vi "Test-TestIntake.vi"() -> ()   [LabVIEW 2023]
doc: "This VI implements the framework and scheduler for your robotics program. It should not be necessary to modify the framework. You are expected to add your code to the VIs called from Robot Main - the ones located in the Team Code folder within the project."
uses:
  <vilib>/Rock Robotics/WPI/DriverStation/WPI_DriverStationRobotMode2.ctl
  Intake/IntakeStates.ctl
  Robot Global Data.vi
  Intake/IntakeCancelSendCmd.vi
  Intake/IntakeAlgaeSendCmd.vi
  Intake/IntakeDepositAlgaeSendCmd.vi
  Intake/IntakeCoralSendCmd.vi
  Intake/IntakeDepositCoralSendCmd.vi
  <vilib>/Rock Robotics/WPI/ThirdParty/JAS_Junk/TrajLib/Trajectory_Library.lvlib
panel:
  out "Numeric":i32
  out "CurrentState":T1
  in  "HaveAlgae":bool
  in  "HaveCoral":bool
  out "Waveform Chart":T2(graph)
  out "Right Motor Out":dbl format="%9.1f"
  in  "IntakeCoral":bool
  in  "CmdSpecific":bool
  in  "Specific":dbl
  in  "IntakeAlgae":bool
  out "Left Motor Out":dbl format="%9.1f"
  in  "DepositCoral":bool
  in  "DepositAlgae":bool
  in  "Canel":bool
  out "Robot Mode":T3
  out "Top Motor Out":dbl format="%9.2f"
  in  "error in (no error)":errorcluster
  in  "Finish":bool
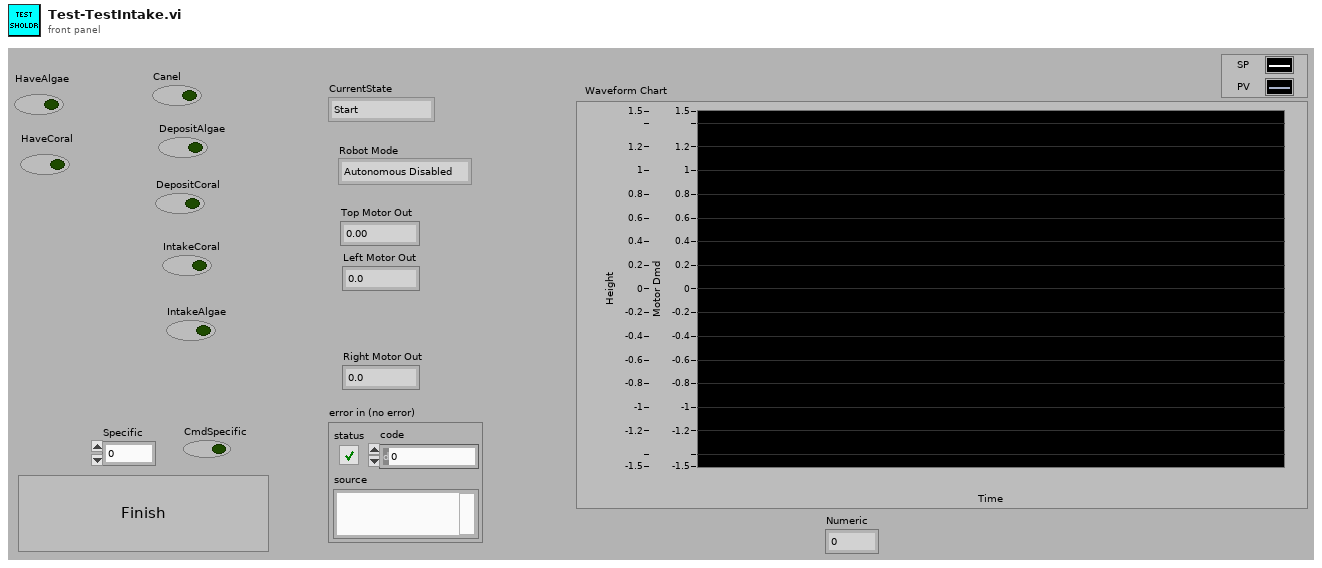
[diagram p1: front panel]
types:
  T1 = typedef "IntakeStates.ctl" = enum16{"Start", "WaitForCommand", "IntakeCoral", "IntakeAlgae", "WaitForCoral", "WaitForAlgae", "DepositCoral", "DepositAlgae", "DepositCoralTimer", "DepositAlgaeTimer"}
  T2 = cluster{"ElevatorPosDemandHeight":dbl, "ElevHeightInch":dbl, "MotorDemand":dbl}
  T3 = typedef "WPI_DriverStationRobotMode2.ctl" = enum16{"Autonomous Disabled", "Autonomous Enabled", "Teleop Disabled", "Teleop Enabled", "Disconnected", "Finish", "Test Disabled", "Test Enabled", "Emergency Stopped"}
  T4 = cluster{"MotorDemandTop":dbl, "MotorDemandLeft":dbl, "MotorDemandRight":dbl}
  T5 = typedef "WPI_DriverStationMatch Info.ctl" = cluster{"Autonomous Elapsed Seconds":dbl, "TeleOp Elapsed Seconds":dbl, "Disabled Elapsed Seconds":dbl, "Visited Autonomous":bool, "Visited TeleOp":bool, "Visited Disabled":bool, "Autonomous Settings":cluster{"Autonomous Style":enum16{"Iterative", "Independent"}, "VI Refnum":refnum<vi>}}
  T6 = typedef "WPI_DriverStationDerivedRobotMode.ctl" = enum16{"Init", "Execute", "Stop"}
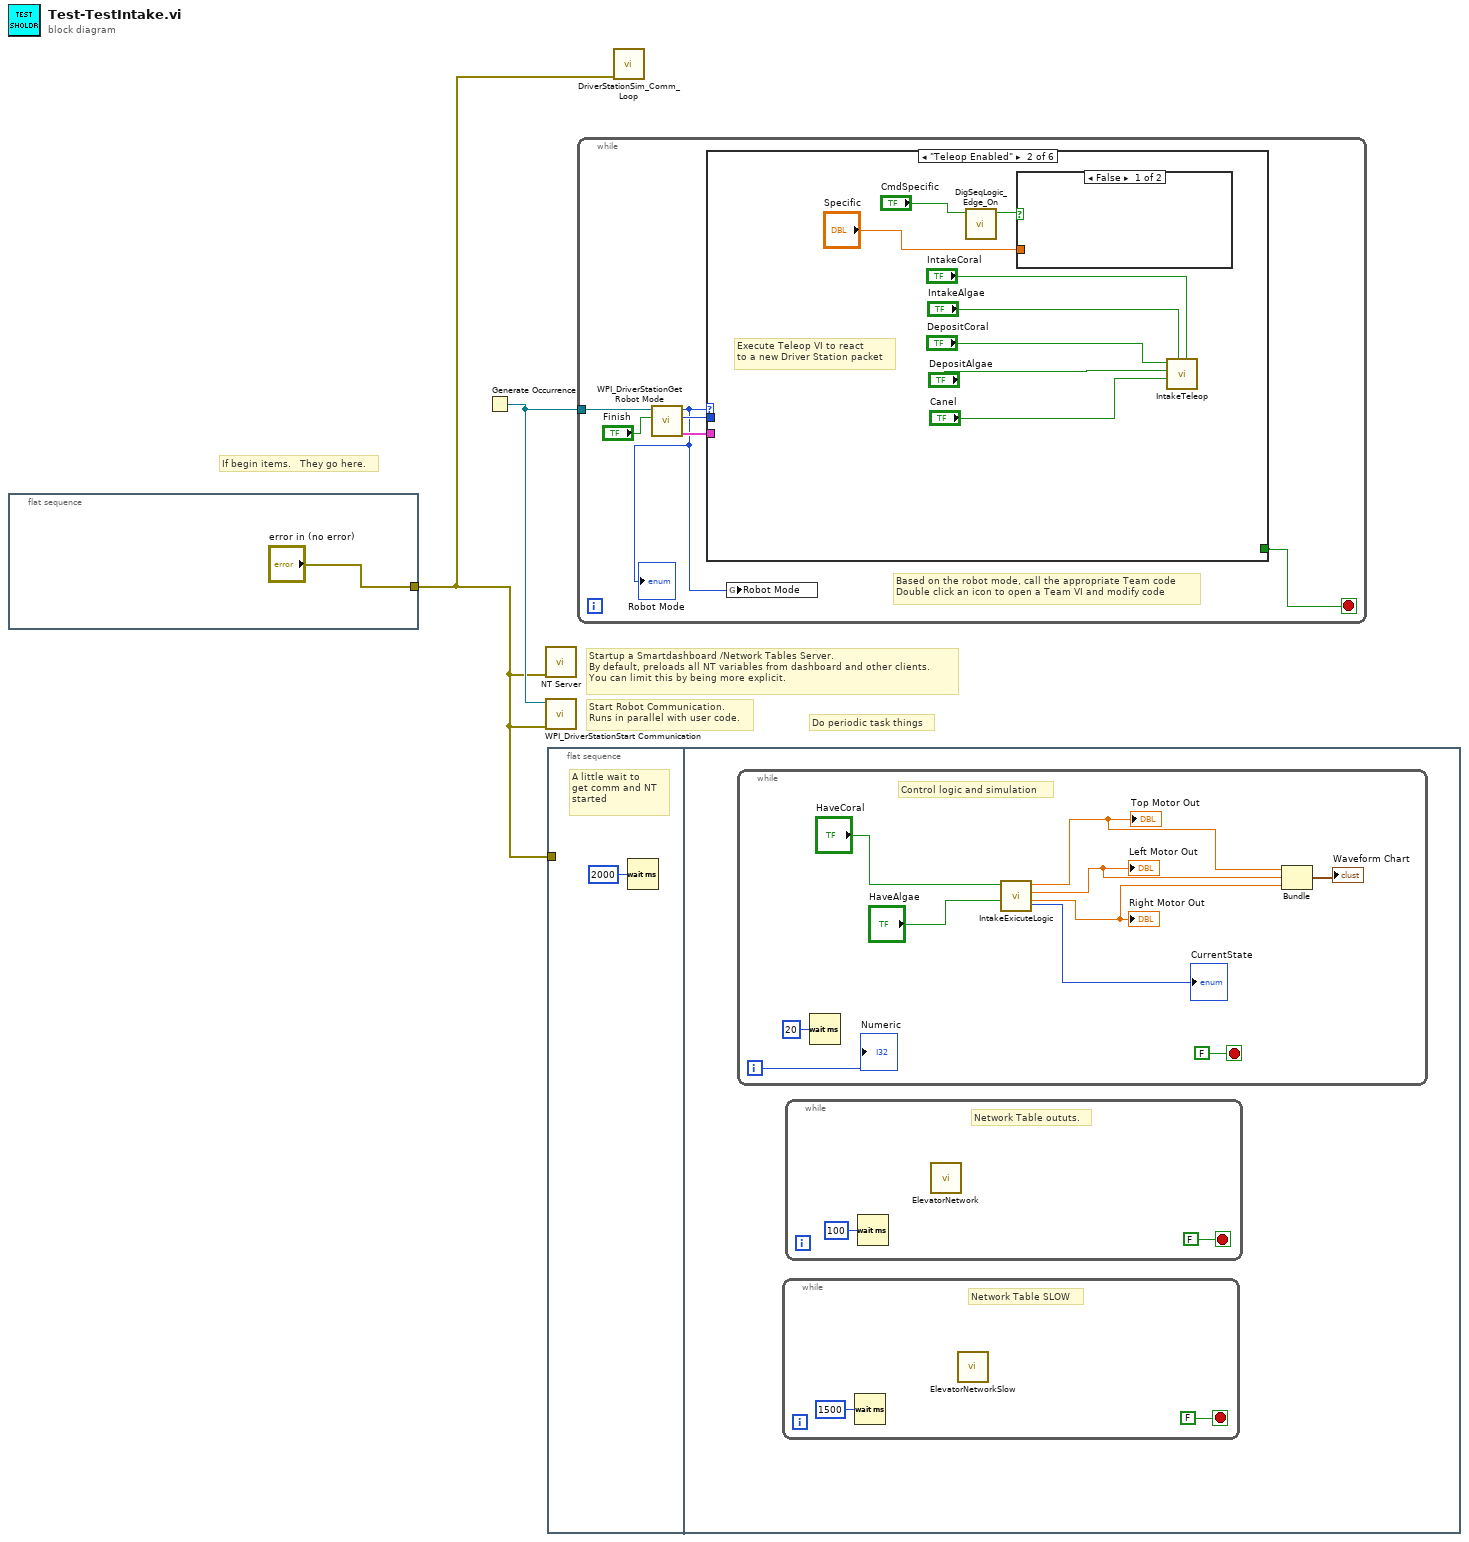
[diagram p0: block diagram]
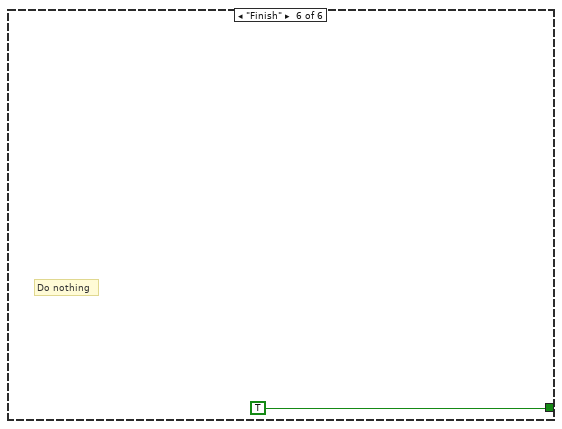
[diagram p7: hidden frame]
diagram:
  # "If begin items.   They go here."
  # "Do periodic task things"
  # "Startup a Smartdashboard /Network Tables Server.\nBy default, preloads all NT variables from dashboard and other clients.\nYou can limit this by being more explicit."
  # "Start Robot Communication.\nRuns in parallel with user code."
  n1 = flat-sequence {
    tunnel: ["error in (no error)"] -> w1
    frame #0 {
    }
  }
  n2 = Generate Occurrence() -> (w2:refnum<k4>)
  n3 = call <vilib>:"NT Server.vi"("error in (no error)"=w1) -> ()  [unwired: 10 in, 1 out]
  n4 = call <vilib>:"WPI_DriverStationStart Communication.vi"("error in (no error)"=w1, "occurrence"=w2) -> ()  [unwired: 1 in, 9 out]
  n5 = flat-sequence {
    tunnel: w1 -> [_]
    frame #0 {
      # "A little wait to\nget comm and NT\nstarted"
      n6 = Wait (ms)(milliseconds to wait=u32 2000) -> ()  [unwired: 1 out]
    }
    frame #1 {
      n7 = while {
        i -> [w9]
        stop <- FALSE stop-if-true
        # "Control logic and simulation"
        n8 = Wait (ms)(milliseconds to wait=u32 20) -> ()  [unwired: 1 out]
        n9 = call "IntakeExicuteLogic.vi"("HaveAlgae"="HaveAlgae", "HaveCoral"="HaveCoral") -> ("MotorDemandRight"=w12:dbl, "MotorDemandLeft"=w13:dbl, "MotorDemandTop"=w14:dbl, "CurrentState"=→"CurrentState":T1)  [unwired: 6 in]
        "Top Motor Out" <- w14
        "Left Motor Out" <- w13
        "Right Motor Out" <- w12
        n10 = Bundle("MotorDemandTop"=w14, "MotorDemandLeft"=w13, "MotorDemandRight"=w12) -> (→"Waveform Chart":T4)  [unwired: 1 in]
        "Numeric" <- w9
      }
      n11 = while {
        stop <- FALSE stop-if-true
        # "Network Table SLOW"
        n12 = Wait (ms)(milliseconds to wait=u32 1500) -> ()  [unwired: 1 out]
        n13 = call "ElevatorNetworkSlow.vi"() -> ()  [unwired: 11 in, 1 out]
      }
      n14 = while {
        stop <- FALSE stop-if-true
        # "Network Table oututs."
        n15 = Wait (ms)(milliseconds to wait=u32 100) -> ()  [unwired: 1 out]
        n16 = call "ElevatorNetwork.vi"() -> ()  [unwired: 11 in, 1 out]
      }
    }
  }
  n17 = while {
    tunnel: w2 -> [w24]
    stop <- w19 stop-if-true
    # "Based on the robot mode, call the appropriate Team code\nDouble click an icon to open a Team VI and modify code"
    n18 = call <vilib>:"WPI_DriverStationGet Robot Mode.vi"("Finish"="Finish", "DS Occurrence"=w24) -> ("Match Info out"=w21:T5, "Call Context"=w23:T6, "Robot Mode"=w20:T3)  [unwired: 7 out]
    "Robot Mode" <- w20
    n19 = case shown="\"Teleop Enabled\"" w20 {
      tunnel: w23 -> [_ _ _ _ _ _]
      tunnel: w21 -> [_ _ _ _ _ _]
      tunnel: [_ _ _ _ _ TRUE] -> w19
      frame "Autonomous Enabled" {
        # "Do nothing...."
      }
      frame "Teleop Enabled" {
        # "Execute Teleop VI to react\nto a new Driver Station packet"
        n20 = call <vilib>:"DigSeqLogic_Edge_On.vi"("Input"="CmdSpecific") -> ("On Edge"=w32:bool)  [unwired: 10 in]
        n21 = case shown="False" w32 {
          tunnel: "Specific" -> [_ _]
          frame False {
          }
          frame True {
          }
        }
        n22 = call "IntakeTeleop.vi"("CmdIntakeCoral"="IntakeCoral", "CmdIntakeAlgae"="IntakeAlgae", "CmdIntakeCancel"="Canel", "CmdIntakeDepositAlgae"="DepositAlgae", "CmdIntakeDepositCoral"="DepositCoral") -> ()  [unwired: 7 in]
      }
      frame "Test Disabled", "Test Enabled" {
        # "Do nothing"
      }
      frame "Autonomous Disabled", "Teleop Disabled" {
        # "Do nothing."
      }
      frame "Disconnected", Default {
        # "Driver Station packet didn't arrive.\nPossibly useful for diagnostics"
      }
      frame "Finish" {
        # "Do nothing"
      }
    }
    n23 = global write "Robot Global Data.vi" "Robot Mode"(w20) -> ()
  }
  n24 = call <vilib>:"DriverStationSim_Comm_Loop.vi"("error in (no error)"=w1) -> ()  [unwired: 11 in]
